vi "svx_Polar_Property_Dialog_Cancel.vi"(6 "Plot Legend ref in":refnum<vi>, 8 "Cursor Info ref in":refnum<vi>, 9 "z scale graph ref in":refnum<vi>, 10 "Polar Plot ref in":refnum<vi>, 11 "State in":T1={"Property Name"=[], "Container bounds"={"Width"=550, "Height"=250}, "Scale range"={"Maximum"=1.0, "Increment"=1.0}, "PointIdx"=0, "Marker list"=[], "Color settings"={"Arrow color"=16860, "Magnitude major grid"=13816530, "Magnitude minor grid"=16777216, "Phase grid"=13816530, "Phase scale marker text"=0}, "Magnitude scale name"="Magnitude", "Magnitude scale format string"="%#.2e", "MagnitudeScale:Visible"=TRUE, "MagnitudeScaleLabel:Visible"=TRUE, "PhaseScale:Visible"=TRUE, "Marker:Visible"=TRUE, "Cursor:Visible"=FALSE, "CursorName:Visible"=TRUE, "Autoscale"=TRUE, "Marker color"=16860, "Line color"=16711680, "Cursor color"=16711680, "Magnitude scale marker color"=0, "Plot.Line Style"=0, "Plot.Line Width"=0, "Plot.Point Style"=0, "Cursor.Line Style"=0, "Cursor.Line Width"=0, "Cursor.Point Style"=0, "Cursor.Style"=4, "Marker.Point Style"=2, "Point/fill color"=16711680, "Background color"=16777225, "Cursor name"="", "Cursor Release"=refnum, "Scale Range Change"=refnum, "data size(s)"=[], "Selectors:Visible"=TRUE, "Selector:ring Strings"={"Selector:Custom Strings"=FALSE, "Selector:Row Strings []"=[], "Selector:Column Strings []"=[], "User:Row Strings []"=[], "User:Column Strings []"=[]}, "Lock Cursor Info Position"=FALSE, "CursLoc"={"magnitude"=0.0, "phase"=0.0, "time/rev/RPM"=0.0}, "Plot Area:Position"={"Left"=0, "Top"=0}, "Plot Area:Size"={"Width"=0, "Height"=0}, "Marker.Style"=0, "Indication Arcs"=[], "Arc.Selector"=0, "customized marker"=[], "tree Width"=0, " Parents Tags"=[], "Children Tags"=[], "open?"=[], "index"=[{"row index"=0, "column index"=0}], "Label"="", "custom strings changed"=FALSE, "Owning VI"=refnum, "Legend BG color"=16777225, "Legend font color"=0, "column Width"=203, "attribute"=variant} caption="State") -> (3 "State out":T1={"Property Name"=[], "Container bounds"={"Width"=550, "Height"=250}, "Scale range"={"Maximum"=1.0, "Increment"=1.0}, "PointIdx"=0, "Marker list"=[], "Color settings"={"Arrow color"=16860, "Magnitude major grid"=13816530, "Magnitude minor grid"=16777216, "Phase grid"=13816530, "Phase scale marker text"=0}, "Magnitude scale name"="Magnitude", "Magnitude scale format string"="%#.2e", "MagnitudeScale:Visible"=TRUE, "MagnitudeScaleLabel:Visible"=TRUE, "PhaseScale:Visible"=TRUE, "Marker:Visible"=TRUE, "Cursor:Visible"=FALSE, "CursorName:Visible"=TRUE, "Autoscale"=TRUE, "Marker color"=16860, "Line color"=16711680, "Cursor color"=16711680, "Magnitude scale marker color"=0, "Plot.Line Style"=0, "Plot.Line Width"=0, "Plot.Point Style"=0, "Cursor.Line Style"=0, "Cursor.Line Width"=0, "Cursor.Point Style"=0, "Cursor.Style"=4, "Marker.Point Style"=2, "Point/fill color"=16711680, "Background color"=16777225, "Cursor name"="", "Cursor Release"=refnum, "Scale Range Change"=refnum, "data size(s)"=[], "Selectors:Visible"=TRUE, "Selector:ring Strings"={"Selector:Custom Strings"=FALSE, "Selector:Row Strings []"=[], "Selector:Column Strings []"=[], "User:Row Strings []"=[], "User:Column Strings []"=[]}, "Lock Cursor Info Position"=FALSE, "CursLoc"={"magnitude"=0.0, "phase"=0.0, "time/rev/RPM"=0.0}, "Plot Area:Position"={"Left"=0, "Top"=0}, "Plot Area:Size"={"Width"=0, "Height"=0}, "Marker.Style"=0, "Indication Arcs"=[], "Arc.Selector"=0, "customized marker"=[], "tree Width"=0, " Parents Tags"=[], "Children Tags"=[], "open?"=[], "index"=[{"row index"=0, "column index"=0}], "Label"="", "custom strings changed"=FALSE, "Owning VI"=refnum, "Legend BG color"=16777225, "Legend font color"=0, "column Width"=203, "attribute"=variant} caption="State")   [LabVIEW 2017, in "SVX Polar Plot.xctl"]
uses:
  <vilib>/addons/_XControls/Polar Plot/SVX Polar Plot.xctl
  <vilib>/addons/_XControls/Polar Plot/subVIs/svx_Polar_Plot_Internal_State.ctl
  <vilib>/addons/_XControls/Polar Plot/subVIs/svx_Polar_Indication_Arcs.ctl
  <vilib>/addons/_XControls/Polar Plot/subVIs/svx_Polar_Customized_Markers.ctl
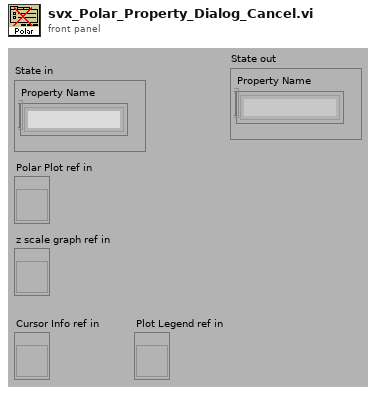
[diagram p1: front panel]
types:
  T1 = typedef "SVX Polar Plot.xctl/svx_Polar_Plot_Internal_State.ctl" = cluster{"Property Name":string[], "Container bounds":cluster{"Width":u32, "Height":u32}, "Scale range":cluster{"Maximum":dbl, "Increment":dbl}, "PointIdx":i32, "Marker list":cluster{"Name":string, "Color":u32, "Style":u8, "Point Style":u8, "Name Visible":bool, "Allow Drag":bool, "Annotation Mode":u32, "Plot":i32, "Index":i32, "Position":cluster{"X":dbl, "Y":dbl}, "X Scale":u32, "Y Scale":u32, "Show Arrow":bool, "Lock Name":bool, "Plot Area":i32, "Label Offset":cluster{"X":dbl, "Y":dbl}}[], "Color settings":cluster{"Arrow color":u32, "Magnitude major grid":u32, "Magnitude minor grid":u32, "Phase grid":u32, "Phase scale marker text":u32}, "Magnitude scale name":string, "Magnitude scale format string":string, "MagnitudeScale:Visible":bool, "MagnitudeScaleLabel:Visible":bool, "PhaseScale:Visible":bool, "Marker:Visible":bool, "Cursor:Visible":bool, "CursorName:Visible":bool, "Autoscale":bool, "Marker color":u32, "Line color":u32, "Cursor color":u32, "Magnitude scale marker color":u32, "Plot.Line Style":i32, "Plot.Line Width":i32, "Plot.Point Style":i32, "Cursor.Line Style":i32, "Cursor.Line Width":i32, "Cursor.Point Style":i32, "Cursor.Style":i32, "Marker.Point Style":i32, "Point/fill color":u32, "Background color":u32, "Cursor name":string, "Cursor Release":refnum<user-event>, "Scale Range Change":refnum<user-event>, "data size(s)":i32[], "Selectors:Visible":bool, "Selector:ring Strings":cluster{"Selector:Custom Strings":bool, "Selector:Row Strings []":string[], "Selector:Column Strings []":string[], "User:Row Strings []":string[], "User:Column Strings []":string[]}, "Lock Cursor Info Position":bool, "CursLoc":cluster{"magnitude":dbl, "phase":dbl, "time/rev/RPM":dbl}, "Plot Area:Position":cluster{"Left":i32, "Top":i32}, "Plot Area:Size":cluster{"Width":u32, "Height":u32}, "Marker.Style":i32, "Indication Arcs":T2, "Arc.Selector":u16, "customized marker":T3, "tree Width":u32, " Parents Tags":string[], "Children Tags":string[], "open?":bool[], "index":cluster{"row index":i32, "column index":i32}[], "Label":string, "custom strings changed":bool, "Owning VI":refnum<vi>, "Legend BG color":u32, "Legend font color":u32, "column Width":u32, "attribute":variant}
  T2 = typedef "SVX Polar Plot.xctl/svx_Polar_Indication_Arcs.ctl" = cluster{"Name":string, "Start radius":dbl, "End radius":dbl, "Line Style":i32, "Line Width":i32, "Border color":u32, "Fill color":u32, "Start angle":i16, "End angle":i16, "Visible":bool}[]
  T3 = typedef "SVX Polar Plot.xctl/svx_Polar_Customized_Markers.ctl" = cluster{"Name":string, "Color":u32, "Style":u8, "Point Style":u8, "Name Visible":bool, "Allow Drag":bool, "Annotation Mode":u32, "Plot":i32, "Index":i32, "Position":cluster{"Magnitude":dbl, "Phase":dbl}, "X Scale":u32, "Y Scale":u32, "Show Arrow":bool, "Lock Name":bool, "Plot Area":i32, "Label Offset":cluster{"Magnitude":dbl, "Phase":dbl}}[]
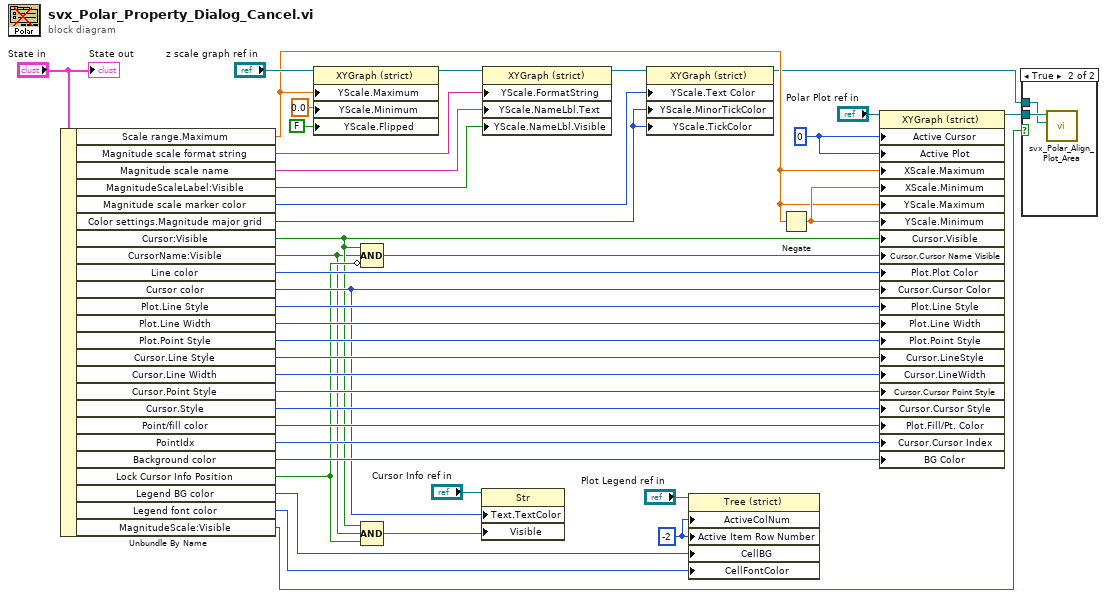
[diagram p0: block diagram]
diagram:
  w17 = -2 ("Active Cell:Active Column Number")
  w39 = u32 0 ("Active Cursor")
  n1 = Unbundle By Name("State in") -> ("Scale range.Maximum"=w8:dbl, "Magnitude scale format string"=w1:string, "Magnitude scale name"=w10:string, "MagnitudeScaleLabel:Visible"=w3:bool, "Magnitude scale marker color"=w7:u32, "Color settings.Magnitude major grid"=w6:u32, "Cursor:Visible"=w13:bool, "CursorName:Visible"=w12:bool, "Line color"=w35:u32, "Cursor color"=w22:u32, "Plot.Line Style"=w32:i32, "Plot.Line Width"=w31:i32, "Plot.Point Style"=w30:i32, "Cursor.Line Style"=w29:i32, "Cursor.Line Width"=w28:i32, "Cursor.Point Style"=w27:i32, "Cursor.Style"=w34:i32, "Point/fill color"=w26:u32, "PointIdx"=w25:i32, "Background color"=w24:u32, "Lock Cursor Info Position"=w20:bool, "Legend BG color"=w16:u32, "Legend font color"=w15:u32, "MagnitudeScale:Visible"=w2:bool)
  n2 = property class="XYGraph (strict)"(reference="z scale graph ref in", "YScale.Maximum"=w8, "YScale.Minimum"=0.0 ("Y Scale.Range:Minimum"), "YScale.Flipped"=FALSE ("Y Scale.Flipped")) -> (reference out=w11:refnum<vi>)  [unwired: 1 in, 1 out]
  n3 = Compound Arithmetic op=AND(w13, w12, invert w20) -> (w19:bool)
  n4 = Compound Arithmetic op=AND(w13, w12, w20) -> (w21:bool)
  n5 = property class="Str"(reference="Cursor Info ref in", "Text.TextColor"=w22, "Visible"=w21) -> ()  [unwired: 1 in, 2 out]
  n6 = property class="XYGraph (strict)"(reference=w11, "YScale.FormatString"=w1, "YScale.NameLbl.Text"=w10, "YScale.NameLbl.Visible"=w3) -> (reference out=w5:refnum<vi>)  [unwired: 1 in, 1 out]
  n7 = property class="XYGraph (strict)"(reference=w5, "YScale.Text Color"=w7, "YScale.MinorTickColor"=w6, "YScale.TickColor"=w6) -> (reference out=w4:refnum<vi>)  [unwired: 1 in, 1 out]
  n8 = property class="Tree (strict)"(reference="Plot Legend ref in", "ActiveColNum"=w17, "Active Item Row Number"=w17, "CellBG"=w16, "CellFontColor"=w15) -> ()  [unwired: 1 in, 2 out]
  n9 = Negate(x=w8) -> (-x=w36:dbl)
  n10 = property class="XYGraph (strict)"(reference="Polar Plot ref in", "Active Cursor"=w39, "Active Plot"=w39, "XScale.Maximum"=w8, "XScale.Minimum"=w36, "YScale.Maximum"=w8, "YScale.Minimum"=w36, "Cursor.Visible"=w13, "Cursor.Cursor Name Visible"=w19, "Plot.Plot Color"=w35, "Cursor.Cursor Color"=w22, "Plot.Line Style"=w32, "Plot.Line Width"=w31, "Plot.Point Style"=w30, "Cursor.LineStyle"=w29, "Cursor.LineWidth"=w28, "Cursor.Cursor Point Style"=w27, "Cursor.Cursor Style"=w34, "Plot.Fill/Pt. Color"=w26, "Cursor.Cursor Index"=w25, "BG Color"=w24) -> (reference out=w33:refnum<vi>)  [unwired: 1 in, 1 out]
  n11 = case shown="True" w2 {
    tunnel: w33 -> [_ w42]
    tunnel: w4 -> [_ w41]
    frame False {
    }
    frame True {
      n12 = call <vilib>:"svx_Polar_Align_Plot_Area.vi"("z scale graph ref in"=w41, "Polar Plot ref in"=w42) -> ()  [unwired: 8 in, 2 out]
    }
  }
  "State out" <- "State in"
